vi "Check That File Exists And Has Correct Extension.vi"(8 "Error In":errorcluster, 10 "Expected File Extension (case insensitive) (e.g \"txt\" or \"EXE\")":string, 11 "Filepath":path) -> (0 "Error Out":errorcluster)   [LabVIEW 2023, in "Error Manager.lvlib"]
uses:
  Error Manager.lvlib
panel:
  # "Input\nInputs to the VI"
  # "Development\nControls or indicators that are useful for development or testing, but which are not outputs of the VI."
  # "Output\nOutputs of the VI"
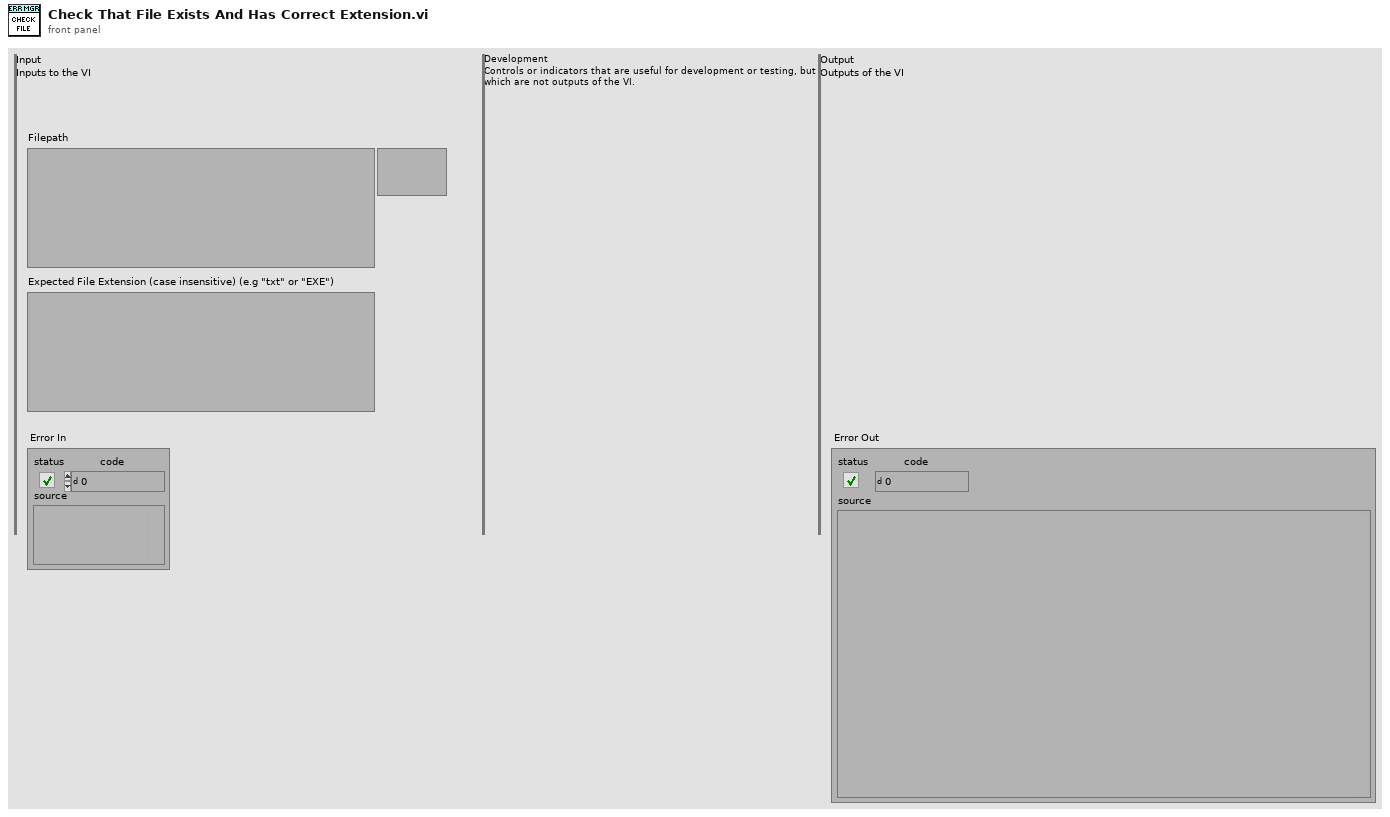
[diagram p1: front panel]
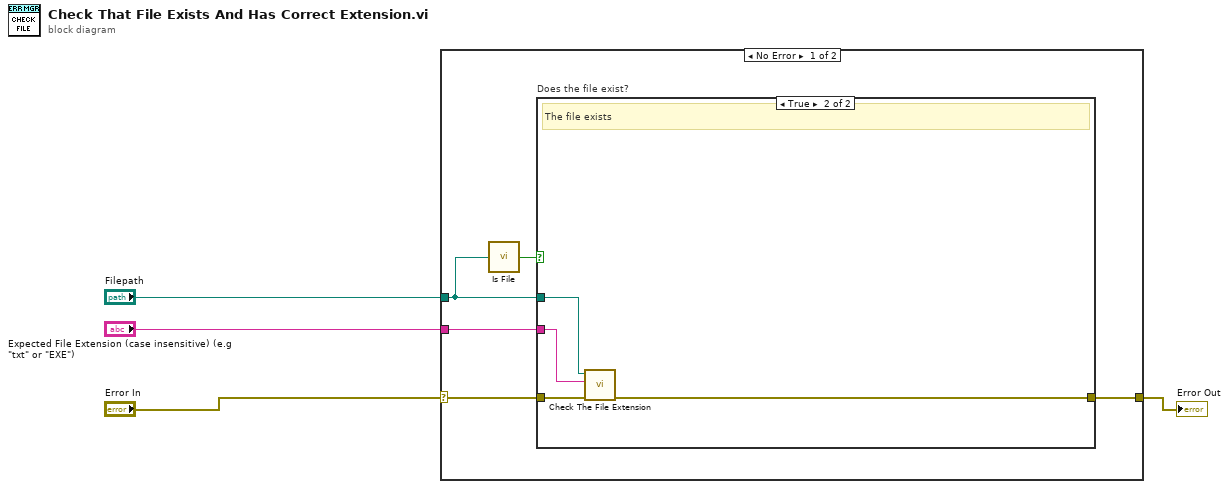
[diagram p0: block diagram]
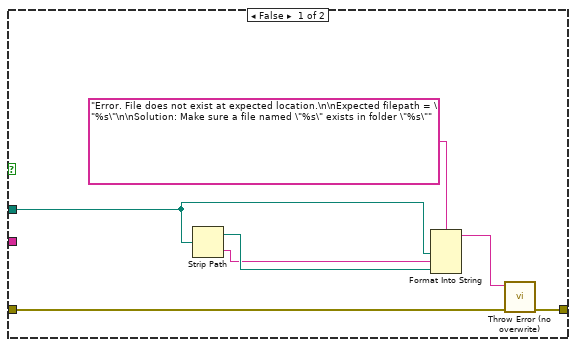
[diagram p2: hidden frame]
diagram:
  n1 = case shown="No Error" "Error In" {
    selector: "Error In" -> [w8 w21]
    tunnel: "Filepath" -> [w6 _]
    tunnel: [w7 w21] -> w2
    tunnel: "Expected File Extension (case insensitive) (e.g \"txt\" or \"EXE\")" -> [w5 _]
    frame No Error {
      n2 = call "Is File.vi"("Input Path"=w6) -> ("Is Existing File?"=w9:bool)
      n3 = case "Does the file exist?" shown="True" w9 {
        tunnel: w8 -> [w12 w20]
        tunnel: [w11 w19] -> w7
        tunnel: w6 -> [w10 w18]
        tunnel: w5 -> [_ w17]
        frame False {
          n4 = Strip Path(path=w10) -> (stripped path=w14:path, name=w13:string)
          n5 = Format Into String(format string="Error. File does not exist at expected location.\n\nExpected filepath = \"%s\"\n\nSolution: Make sure a file named \"%s\" exists in folder \"%s\"", w10, w13, w14) -> (resulting string=w15:string)  [unwired: 2 in, 1 out]
          n6 = call "Throw Error (no overwrite).vi"("error in"=w12, "Error Message (\"\")"=w15) -> ("error out"=w11:errorcluster)  [unwired: 9 in]
        }
        frame True {
          # "The file exists"
          n7 = call "Check The File Extension.vi"("error in"=w20, "Expected File Extension (e.g \"txt\")"=w17, "Filepath"=w18) -> ("error out"=w19:errorcluster)  [unwired: 8 in]
        }
      }
    }
    frame Error {
    }
  }
  "Error Out" <- w2
